vi "Quit Application.vi"(8 "error in (no error)":errorcluster, 11 "JMP application":refnum<k7>) -> (0 "error out":errorcluster)   [LabVIEW 2019, in "JMP Automation.lvlib"]
doc: "Close the JMP application"
uses:
  <instrlib>/LV_JMP_bridge/JMP Automation.lvlib
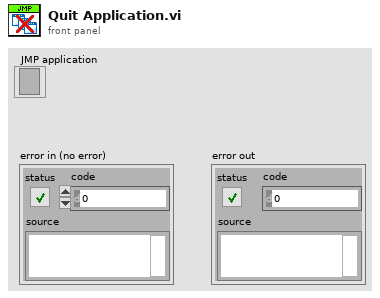
[diagram p1: front panel]
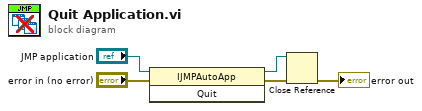
[diagram p0: block diagram]
diagram:
  n1 = invoke class="IJMPAutoApp" method="Quit"(reference="JMP application", error in="error in (no error)") -> (reference out=w1:refnum<k7>, error out=w3:errorcluster)  [unwired: 1 in, 1 out]
  n2 = Close Reference(reference=w1, error in (no error)=w3) -> (error out=→"error out":errorcluster)
